vi "Gather Relevant Data.vi"(11 "Sorted Data":dbl[][](array[numeric])) -> (3 "Array":T1[](array[typedef]))   [LabVIEW 2015]
uses:
  References/Relevant Data.ctl
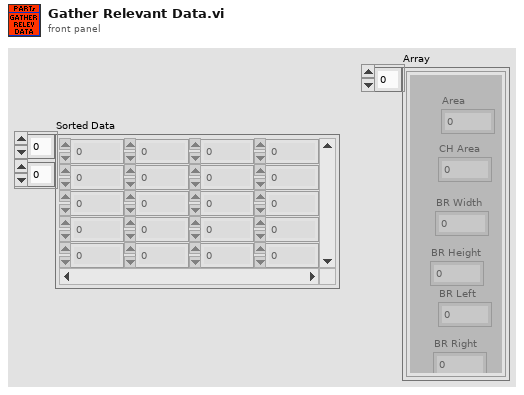
[diagram p1: front panel]
types:
  T1 = typedef "Relevant Data.ctl" = cluster{"Area":dbl, "CH Area":dbl, "BR Width":dbl, "BR Height":dbl, "BR Left":dbl, "BR Right":dbl}
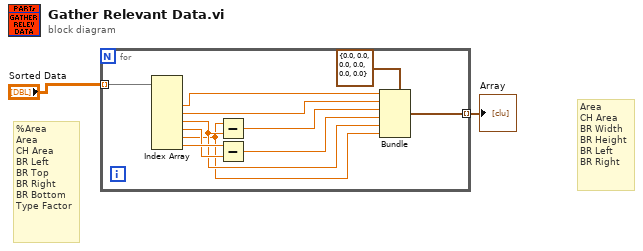
[diagram p0: block diagram]
diagram:
  # "Area\nCH Area\nBR Width\nBR Height\nBR Left\nBR Right"
  # "%Area\nArea\nCH Area\nBR Left\nBR Top\nBR Right\nBR Bottom\nType Factor"
  n1 = for {
    tunnel: "Sorted Data" -> [w11] mode=indexing
    tunnel: [w6] -> w1 mode=indexing
    n2 = Index Array(array=w11) -> (element #2=w13:dbl, element #3=w12:dbl, element #4=w5:dbl, element #5=w9:dbl, element #6=w4:dbl, element #7=w10:dbl)  [unwired: 7 in, 1 out]
    n3 = Subtract(x=w4, y=w5) -> (x-y=w8:dbl)
    n4 = Subtract(x=w10, y=w9) -> (x-y=w7:dbl)
    n5 = Bundle(cluster=T1 {"Area"=0.0, "CH Area"=0.0, "BR Width"=0.0, "BR Height"=0.0, "BR Left"=0.0, "BR Right"=0.0} ("Relevant Data"), "Area"=w13, "CH Area"=w12, "BR Width"=w8, "BR Height"=w7, "BR Left"=w5, "BR Right"=w4) -> (w6:T1)
  }
  "Array" <- w1
